vi "PRBS64 Parallel Rx Base.vi"(7 "reset":bool, 9 "input valid":bool=TRUE, 11 "prbs rx":u64) -> (1 "output valid":bool, 3 "pattern mismatch":bool)   [LabVIEW 2023, in "Aurora64b66b Utilities FPGA.lvlib"]
uses:
  Aurora64b66b Utilities FPGA.lvlib
  Program Files/NI/LVAddons/niidl/1/instr.lib/_niInstr/Basic Elements/v1/FPGA/niInstr Basic Elements v1 FPGA.lvlib
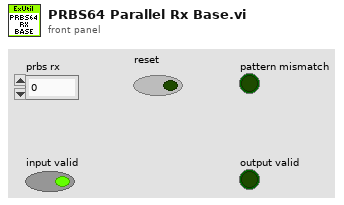
[diagram p1: front panel]
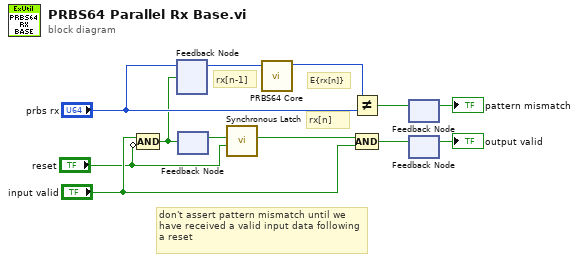
[diagram p0: block diagram]
diagram:
  # "don't assert pattern mismatch until we have received a valid input data following a reset"
  # "rx[n]"
  # "rx[n-1]"
  # "E{rx[n]}"
  n1 = Compound Arithmetic op=AND("input valid", invert "reset") -> (w5:bool)
  n2 = feedback #1() -> (w10:u64)  [unwired: 1 in]
  n3 = feedback-in #1("prbs rx", w5) -> ()
  n4 = feedback #2() -> (w8:bool)  [unwired: 1 in]
  n5 = feedback-in #2(w5) -> ()
  n6 = call "Synchronous Latch.vi"("clear"="reset", "set"=w8) -> ("out"=w7:bool)  [unwired: 9 in]
  n7 = call "PRBS64 Core.vi"("current value"=w10) -> ("next value"=w11:u64)  [unwired: 10 in]
  n8 = Not Equal?(x=w11, y="prbs rx") -> (x != y?=w3:bool)
  n9 = Compound Arithmetic op=AND(w7, "input valid") -> (w2:bool)
  n10 = feedback #3() -> (→"pattern mismatch":bool)  [unwired: 1 in]
  n11 = feedback-in #3(w3) -> ()
  n12 = feedback #4() -> (→"output valid":bool)  [unwired: 1 in]
  n13 = feedback-in #4(w2) -> ()
